vi "Calculate IQ Power Level.vi"(0 "IQ data":cdb[](array[numeric])) -> (4 "power level (dBm)":dbl[](array[numeric]))   [LabVIEW 2013]
doc: "Calculates the power level, in dBm, from the I/Q data."
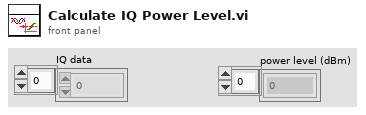
[diagram p1: front panel]
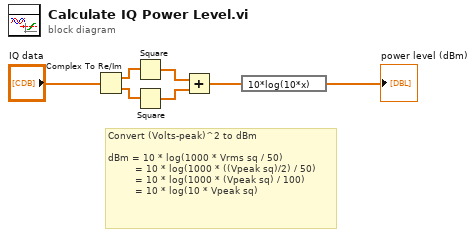
[diagram p0: block diagram]
diagram:
  # "Convert (Volts-peak)^2 to dBm\n\ndBm = 10 * log(1000 * Vrms sq / 50)\n         = 10 * log(1000 * ((Vpeak sq)/2) / 50) \n         = 10 * log(1000 * (Vpeak sq) / 100) \n         = 10 * log(10 * Vpeak sq)"
  n1 = Complex To Re/Im(x + iy="IQ data") -> (x=w6:dbl[], y=w5:dbl[])
  n2 = Square(x=w6) -> (x^2=w4:dbl[])
  n3 = Square(x=w5) -> (x^2=w3:dbl[])
  n4 = Add(x=w4, y=w3) -> (x+y=w2:dbl[])
  n5 = expression code="10*log(10*x)"(w2) -> (→"power level (dBm)":dbl[])
